vi "mlink_enc_read.vi"(8 "error in (no error)":errorcluster, 10 "channel":u8, 11 "connection ID":i32=-1) -> (0 "error out":errorcluster, 1 "position":i32, 2 "direction":enum16{"None", "CW", "CCW"}(ring), 3 "connection ID out":i32)   [LabVIEW 2009, in "MicroDAQ.lvlib" / "mlink.lvlib"]
doc: "This function initializes selected quadrature encoder module (ENC1, ENC2) with provided initial value. The function has to be called before mlink_enc_read() function call."
uses:
  <instrlib>/MicroDAQ/Mlink library wraper/mlink.lvlib
  <instrlib>/MicroDAQ/MLink32.dll
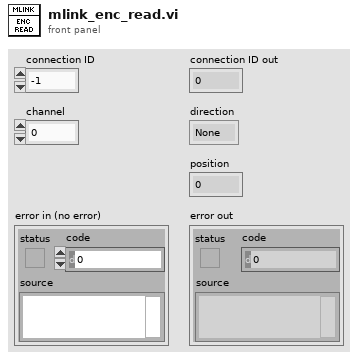
[diagram p1: front panel]
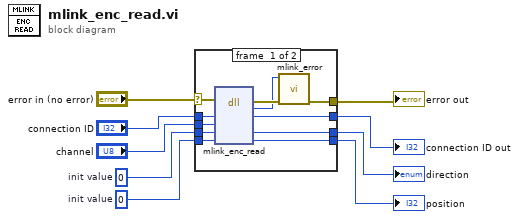
[diagram p0: block diagram]
diagram:
  w4 = u8 0  # init value
  w7 = 0  # init value
  n1 = case shown="No Error" "error in (no error)" {
    selector: "error in (no error)" -> [w16 w24]
    tunnel: "connection ID" -> [w20 w23]
    tunnel: [w19 w23] -> w8
    tunnel: w7 -> [w18 w21]
    tunnel: [w17 w21] -> w6
    tunnel: w4 -> [w15 w22]
    tunnel: [w14 w22] -> w3
    tunnel: "channel" -> [w13 _]
    tunnel: [w10 w24] -> w1
    frame #0 {
      n2 = dll-call lib="C:/Program Files (x86)/National Instruments/LabVIEW 2009/instr.lib/MicroDAQ/MLink32.dll" fn="mlink_enc_read"(error in=w16, "connection ID"=w20, "channel"=w13, "dir"=w15, "position"=w18) -> (error out=w12:errorcluster, "return type"=w11:i32, "connection ID"=w19:i32, "dir"=w14:u8, "position"=w17:i32)  [unwired: 3 in, 1 out]
      n3 = call <instrlib>:"mlink_error.vi"("error in (no error)"=w12, "error code"=w11) -> ("error out"=w10:errorcluster)  [unwired: 9 in]
    }
    frame #1 {
    }
  }
  "connection ID out" <- w8
  "position" <- w6
  "error out" <- w1
  "direction" <- w3
